vi "SPI LM74.vi"(11 "array":u8[](array[numeric])) -> (3 "°C":dbl)   [LabVIEW 2014]
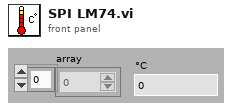
[diagram p1: front panel]
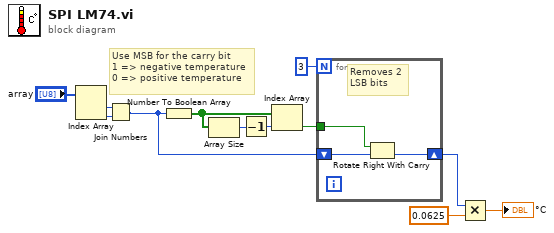
[diagram p0: block diagram]
diagram:
  # "Use MSB for the carry bit\n1 => negative temperature\n0 => positive temperature"
  n1 = Index Array(array="array") -> (element #1=w12:u8, element #2=w11:u8)  [unwired: 2 in]
  n2 = Join Numbers(hi=w12, lo=w11) -> ((hi.lo)=w2:u16)
  n3 = Number To Boolean Array(number=w2) -> (Boolean array=w5:bool[])
  n4 = Array Size(array=w5) -> (size(s)=w4:i32)
  n5 = Decrement(x=w4) -> (x-1=w3:i32)
  n6 = Index Array(array=w5, index=w3) -> (element=w6:bool)
  n7 = for {
    N: 3 -> [_]
    shift-right: [w14] -> w9
    shift-left: w2 -> [w15]
    tunnel: w6 -> [w13]
    # "Removes 2\nLSB bits"
    n8 = Rotate Right With Carry(2:w15, 3:w13) -> (0:w14:u16)  [unwired: 1 out]
  }
  n9 = Multiply(x=w9, y=0.0625) -> (x*y=→"°C":dbl)
